vi "Write 2D Picture ref.vi"(8 "error in (no error)":errorcluster, 10 "2D Picture ref":refnum<vi>, 11 "class2 in":refnum<class "class2.lvclass">) -> (0 "error out":errorcluster, 3 "class2 out":refnum<class "class2.lvclass">)   [LabVIEW 2013, in "class2.lvclass"]
uses:
  class2.lvclass
  class2.lvclass/class2.ctl
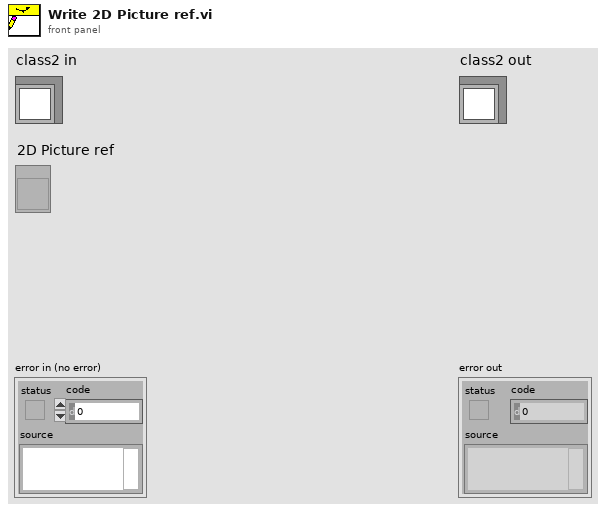
[diagram p1: front panel]
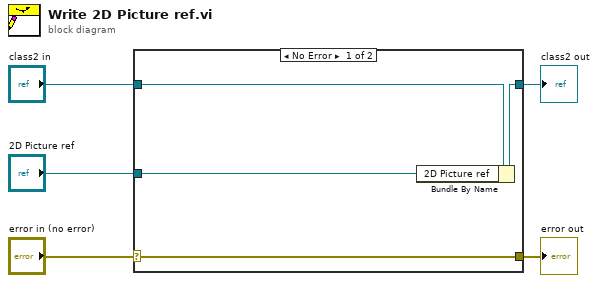
[diagram p0: block diagram]
diagram:
  n1 = case shown="No Error" "error in (no error)" {
    selector: "error in (no error)" -> [w9 w10]
    tunnel: [w9 w10] -> w4
    tunnel: [w7 w11] -> w2
    tunnel: "class2 in" -> [w8 w11]
    tunnel: "2D Picture ref" -> [w6 _]
    frame No Error {
      n2 = Bundle By Name(cluster=w8, "2D Picture ref"=w6) -> (w7:refnum<class "class2.lvclass">)
    }
    frame Error {
    }
  }
  "error out" <- w4
  "class2 out" <- w2
